vi "Select chan.vi"(10 "Channel":string, 11 "output cluster":T1) -> (3 "Output":dbl)   [LabVIEW 2023]
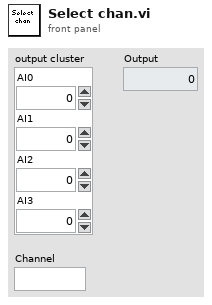
[diagram p1: front panel]
types:
  T1 = cluster{"AI0":dbl, "AI1":dbl, "AI2":dbl, "AI3":dbl}
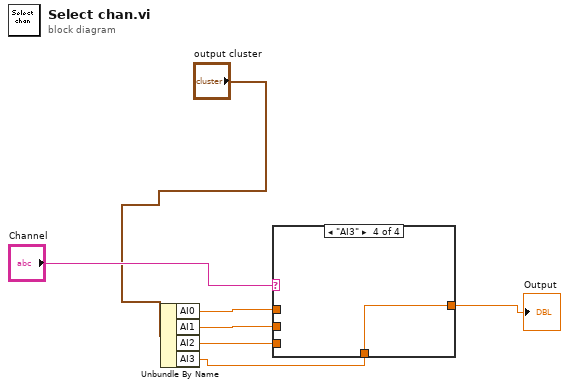
[diagram p0: block diagram]
diagram:
  n1 = Unbundle By Name("output cluster") -> ("AI0"=w4:dbl, "AI1"=w5:dbl, "AI2"=w6:dbl, "AI3"=w7:dbl)
  n2 = case shown="\"AI3\"" "Channel" {
    tunnel: [w8 w9 w10 w11] -> w3
    tunnel: w4 -> [w8 _ _ _]
    tunnel: w5 -> [_ w9 _ _]
    tunnel: w6 -> [_ _ w10 _]
    tunnel: w7 -> [_ _ _ w11]
    frame "AI0", Default {
    }
    frame "AI1" {
    }
    frame "AI2" {
    }
    frame "AI3" {
    }
  }
  "Output" <- w3
